vi "TDMS Advanced Synchronous Read Speed Test.vi"() -> ()   [LabVIEW 2023]
doc: "This example demonstrates how to benchmark the streaming performance when you use the TDMS Advanced Synchronous Read function to read data from a .tdms file. This VI measures the time it takes to continuously read data from a file and calculates the average data throughput in bytes/second."
panel:
  in  "Disable Buffering? (T)":bool=TRUE
  out "Bytes/second":dbl format="%#_4p"
  out "Current Number of Reads":i32
  out "Total Number of Reads":u64
  in  "Read Block Size (bytes)":u64=4194304 step=1048576
  # "Overview: Demonstrates how to benchmark the streaming performance when you use the TDMS Advanced Synchronous Read function to read data from a .tdms file. \nInstructions:\n1. Make sure you have already run TDMS Advanced Synchronous Write Speed Test.vi.\n2. Run the VI.\n3. Delete the TDMS file (located at [LabVIEW Data]\\Example TDMS Synchronous Speed Test Data.tdms) when you are done."
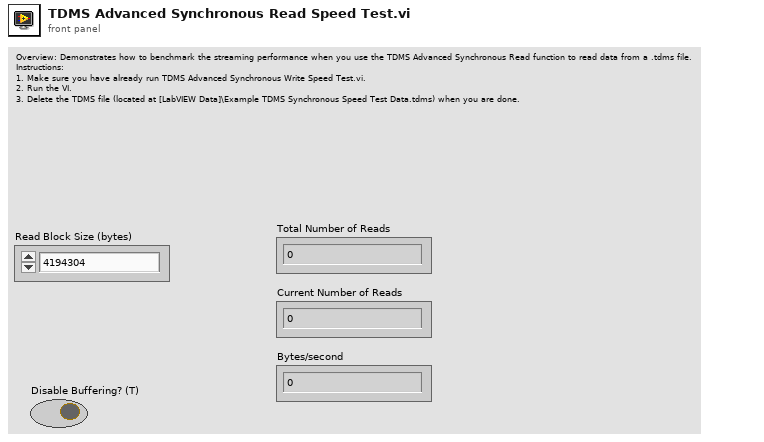
[diagram p1: front panel]
types:
  T1 = enum16{"open", "open or create", "create or replace", "create", "open (read-only)"}
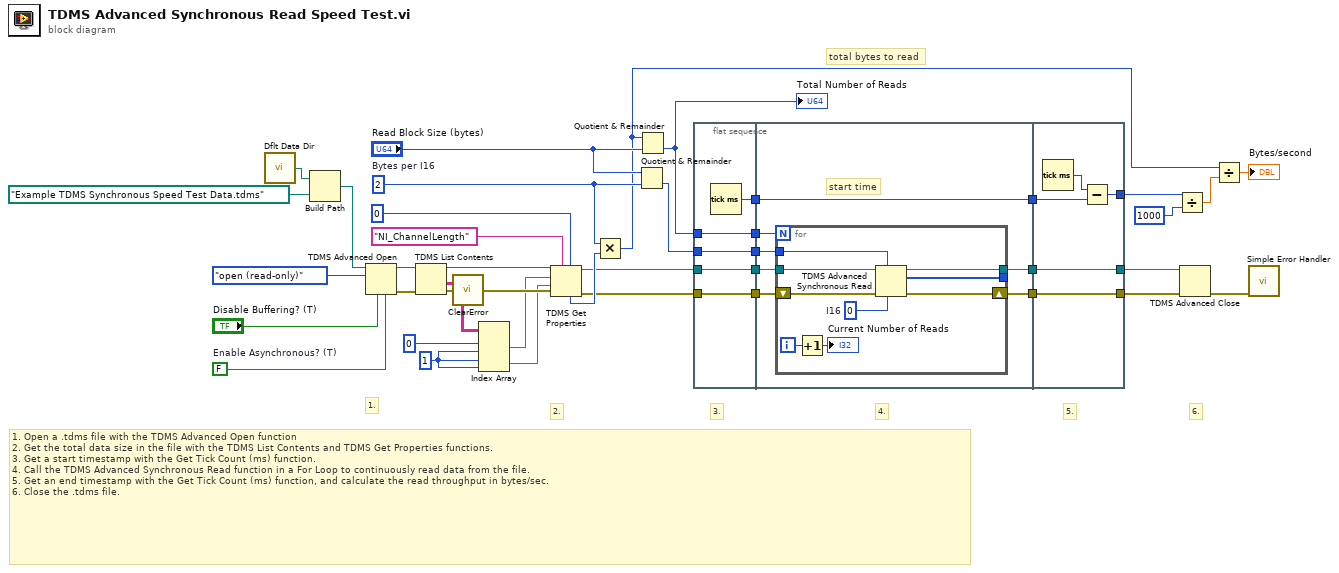
[diagram p0: block diagram]
diagram:
  w23 = 1 ("disabled index (col)")
  w30 = FALSE  # Enable Asynchronous? (T)
  w15 = u64 2  # Bytes per I16
  # "total bytes to read"
  # "6."
  # "2."
  # "5."
  # "4."
  # "3."
  # "1."
  # "1. Open a .tdms file with the TDMS Advanced Open function \n2. Get the total data size in the file with the TDMS List Contents and TDMS Get Properties functions. \n3. Get a start timestamp with the Get Tick Count (ms) function.\n4. Call the TDMS Advanced Synchronous Read function in a For Loop to continuously read data from the file.\n5. Get an end timestamp with the Get Tick Count (ms) function, and calculate the read throughput in bytes/sec.\n6. Close the .tdms file."
  n1 = call <vilib>:"Dflt Data Dir.vi"() -> ("App:Default Data Directory"=w2:path)
  n2 = Build Path(base path=w2, name or relative path=path "Example TDMS Synchronous Speed Test Data.tdms") -> (appended path=w3:path)
  n3 = TDMS Advanced Open(4:w30, 6:"Disable Buffering? (T)", 10:T1."open (read-only)" ("Operation"), 11:w3) -> (0:w26:errorcluster, 3:w27:refnum<k34>)  [unwired: 1 in, 1 out]
  n4 = TDMS List Contents(4:w26, 7:w27) -> (0:w1:errorcluster, 1:w25:string[][], 3:w21:refnum<k34>)  [unwired: 1 in, 1 out]
  n5 = call <vilib>:"ClearError.vi"("error in (no error)"=w1) -> ("error out"=w22:errorcluster)
  n6 = Index Array(array=w25, index (row) #1=0 ("index (row)"), index (col) #1=w23, index (row) #2=w23, index (col) #2=w23) -> (element #1=w20:string, element #2=w19:string)
  n7 = TDMS Get Properties(5:0, 7:"NI_ChannelLength" ("property name"), 8:w22, 9:w19, 10:w20, 11:w21) -> (0:w13:errorcluster, 3:w11:refnum<k34>, 4:w16:i32)  [unwired: 3 out]
  n8 = Multiply(x=w15, y=w16) -> (x*y=w6:u64)
  n9 = Quotient & Remainder(x="Read Block Size (bytes)", y=w15) -> (floor(x/y)=w28:u64)  [unwired: 1 out]
  n10 = Quotient & Remainder(x=w6, y="Read Block Size (bytes)") -> (floor(x/y)=w5:u64)  [unwired: 1 out]
  "Total Number of Reads" <- w5
  n11 = flat-sequence {
    tunnel: [w46] -> w41
    tunnel: w5 -> [w45]
    tunnel: [w45] -> w40
    tunnel: [w44] -> w29
    tunnel: w28 -> [w44]
    tunnel: [w43] -> w14
    tunnel: w13 -> [w43]
    tunnel: [w42] -> w12
    tunnel: w11 -> [w42]
    tunnel: w41 -> [w53]
    tunnel: [w53] -> w39
    tunnel: [w52] -> w38
    tunnel: [w51] -> w37
    tunnel: w40 -> [w50]
    tunnel: w29 -> [w49]
    tunnel: w14 -> [w48]
    tunnel: w12 -> [w47]
    tunnel: w39 -> [w66]
    tunnel: w38 -> [w65]
    tunnel: [w65] -> w35
    tunnel: [w64] -> w34
    tunnel: w37 -> [w64]
    tunnel: [w63] -> w7
    frame #0 {
      n12 = Tick Count (ms)() -> (millisecond timer value=w46:u32)
    }
    frame #1 {
      # "start time"
      n13 = for {
        N: w50 -> [_]
        tunnel: [w58] -> w52
        shift-right: [w62] -> w51
        shift-left: w48 -> [w61]
        tunnel: [w57] -> _
        tunnel: w49 -> [w55]
        tunnel: w47 -> [w54]
        i -> [w60]
        w56 = i16 0  # I16
        n14 = Increment(x=w60) -> (x+1=→"Current Number of Reads":i32)
        n15 = TDMS Advanced Synchronous Read(6:w56, 7:w55, 8:w61, 11:w54) -> (0:w62:errorcluster, 2:w57:i16[], 3:w58:refnum<k34>)  [unwired: 1 out]
      }
    }
    frame #2 {
      n16 = Tick Count (ms)() -> (millisecond timer value=w67:u32)
      n17 = Subtract(x=w67, y=w66) -> (x-y=w63:u32)
    }
  }
  n18 = Divide(x=w7, y=u32 1000) -> (x/y=w9:dbl)
  n19 = TDMS Advanced Close(8:w34, 11:w35) -> (0:w36:errorcluster)  [unwired: 2 in, 1 out]
  n20 = Divide(x=w6, y=w9) -> (x/y=→"Bytes/second":dbl)
  n21 = call <vilib>:"Simple Error Handler.vi"("error in (no error)"=w36) -> ()  [unwired: 1 in, 8 out]
